vi "Pre Launch Init.vi"(11 "Test Actor in":refnum<class "Example Actor.lvclass">) -> (0 "error out":errorcluster, 3 "Test Actor out":refnum<class "Example Actor.lvclass">)   [LabVIEW 2017, in "Example Actor.lvlib" / "Example Actor.lvclass"]
doc: "Sends a high priority message to it's self to notify the monitor that it's spawned. If it's in the runtime environment, this message is never sent, meaning the monitor will never spawn\n\nCopyright: MGI\n\nAuthored by Derek Trepanier\nsupport@mooregoodideas.com\nwww.mooregoodideas.com\n\nCopyright (c) 2014, Moore Good Ideas, Inc.\n\nAll rights reserved.\n\nRedistribution and use in source and binary forms, with or without modification, are permitted provided that the following conditions are met:\n\n * Redistributions of source code must retain the above copyright notice, this list of conditions and the following disclaimer.\n * Redistributions in binary form must reproduce the above copyright notice, this list of conditions and the following disclaimer in the documentation and/or other materials provided with the distribution.\n * Neither the name of Moore Good Ideas, Inc. nor the names of its contributors may be used to endorse or promote products derived from this software without specific prior written permission.\n\nTHIS SOFTWARE IS PROVIDED BY THE COPYRIGHT HOLDERS AND CONTRIBUTORS \"AS IS\" AND ANY EXPRESS OR IMPLIED WARRANTIES, INCLUDING, BUT NOT LIMITED TO, THE IMPLIED WARRANTIES OF MERCHANTABILITY AND FITNESS FOR A PARTICULAR PURPOSE ARE DISCLAIMED. IN NO EVENT SHALL THE COPYRIGHT OWNER OR CONTRIBUTORS BE LIABLE FOR ANY DIRECT, INDIRECT, INCIDENTAL, SPECIAL, EXEMPLARY, OR CONSEQUENTIAL DAMAGES (INCLUDING, BUT NOT LIMITED TO, PROCUREMENT OF SUBSTITUTE GOODS OR SERVICES; LOSS OF USE, DATA, OR PROFITS; OR BUSINESS INTERRUPTION) HOWEVER CAUSED AND ON ANY THEORY OF LIABILITY, WHETHER IN CONTRACT, STRICT LIABILITY, OR TORT (INCLUDING NEGLIGENCE OR OTHERWISE) ARISING IN ANY WAY OUT OF THE USE OF THIS SOFTWARE, EVEN IF ADVISED OF THE POSSIBILITY OF SUCH DAMAGE."
uses:
  Example Actor.lvclass
  D:/software/LabView_MonitoredActor/monitored-actor-core/Source/Monitored Actor/Monitored Actor/Monitored Actor.lvclass
  Example Actor.lvclass/Example Actor.ctl
  monitored-actor-core/Source/Monitored Actor/Monitored Actor/Monitored Actor.lvclass
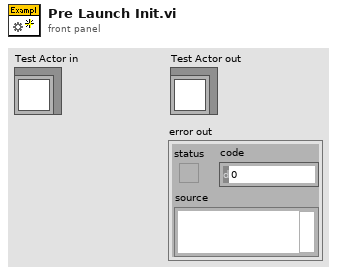
[diagram p1: front panel]
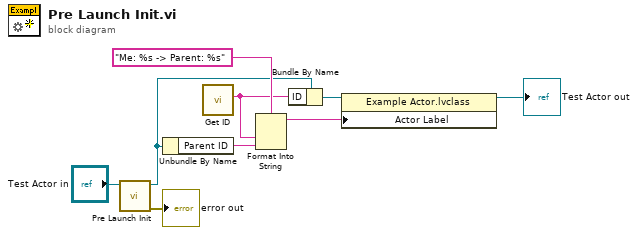
[diagram p0: block diagram]
diagram:
  n1 = call-parent "Pre Launch Init.vi"("Monitored Actor in"="Test Actor in") -> ("error out"=→"error out":errorcluster, "Monitored Actor out"=w2:refnum<class "Example Actor.lvclass">)  [unwired: 9 in]
  n2 = Unbundle By Name(w2) -> ("Parent ID"=w6:string)
  n3 = call "Get ID.vi"() -> ("ID"=w5:string)  [unwired: 11 in]
  n4 = Format Into String(format string="Me: %s -> Parent: %s", w5, w6) -> (resulting string=w4:string)  [unwired: 2 in, 1 out]
  n5 = Bundle By Name(cluster=w2, "ID"=w5) -> (w8:refnum<class "Example Actor.lvclass">)
  n6 = property class="Example Actor.lvclass"(reference=w8, "Actor Label"=w4) -> (reference out=→"Test Actor out":refnum<class "Example Actor.lvclass">)  [unwired: 1 in, 1 out]
